vi "Write to TDMS File.vi"(7 "Track Name":string, 8 "Error In":errorcluster, 9 "Write Position":i64, 10 "Audio In":T1, 11 "TDMS Reference In":refnum<k34>) -> (0 "Error Out":errorcluster, 3 "TDMS Reference Out":refnum<k34>)   [LabVIEW 2014]
doc: "Write to a TDMS File. You can specify a Track Name, write position, and data to write."
uses:
  Controls/Audio In.ctl
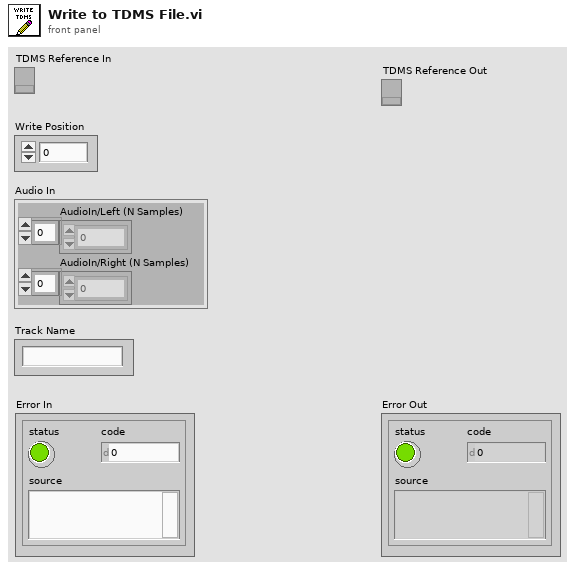
[diagram p1: front panel]
types:
  T1 = typedef "Audio In.ctl" = cluster{"AudioIn/Left (N Samples)":i16[], "AudioIn/Right (N Samples)":i16[]}
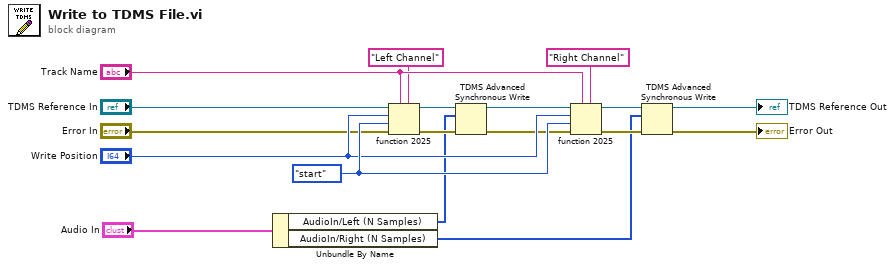
[diagram p0: block diagram]
diagram:
  w16 = enum16{"start", "end"}."start" ("from (0:start)")
  n1 = Unbundle By Name("Audio In") -> ("AudioIn/Left (N Samples)"=w3:i16[], "AudioIn/Right (N Samples)"=w2:i16[])
  n2 = fn#2025(5:"Left Channel" ("channel name in"), 7:"Track Name", 8:"Error In", 9:w16, 10:"Write Position", 11:"TDMS Reference In") -> (0:w9:errorcluster, 3:w10:refnum<k34>)
  n3 = TDMS Advanced Synchronous Write(8:w9, 10:w3, 11:w10) -> (0:w1:errorcluster, 3:w4:refnum<k34>)
  n4 = fn#2025(5:"Right Channel" ("channel name in"), 7:"Track Name", 8:w1, 9:w16, 10:"Write Position", 11:w4) -> (0:w6:errorcluster, 3:w7:refnum<k34>)
  n5 = TDMS Advanced Synchronous Write(8:w6, 10:w2, 11:w7) -> (0:→"Error Out":errorcluster, 3:→"TDMS Reference Out":refnum<k34>)
